vi "StopTrigger.vi"(8 "error in (no error)":errorcluster, 10 "trigger":string, 11 "PredictiveMaintenance in":refnum<class "PredictiveMaintenance.lvclass">) -> (0 "error out":errorcluster, 3 "PredictiveMaintenance out":refnum<class "PredictiveMaintenance.lvclass">)   [LabVIEW 2019, in "PredictiveMaintenance.lvlib" / "PredictiveMaintenance.lvclass"]
uses:
  PredictiveMaintenance.lvclass
  PredictiveMaintenance.lvclass/PredictiveMaintenance.ctl
  typedefs/Trigger_Data.ctl
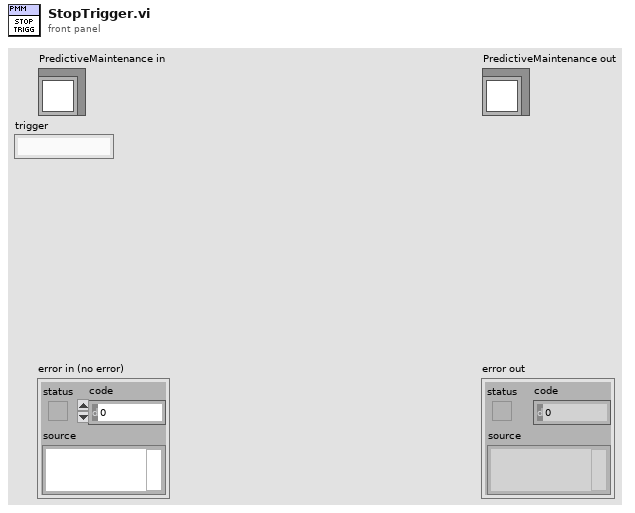
[diagram p1: front panel]
types:
  T1 = typedef "PredictiveMaintenance.lvlib/PredictiveMaintenance.lvclass/Trigger_Data.ctl" = cluster{"trigger":string, "curr_val (h)":dbl, "warn_limit (h)":dbl, "err_limit (h)":dbl, "running_timestamp":timestamp, "counter (h)":dbl}
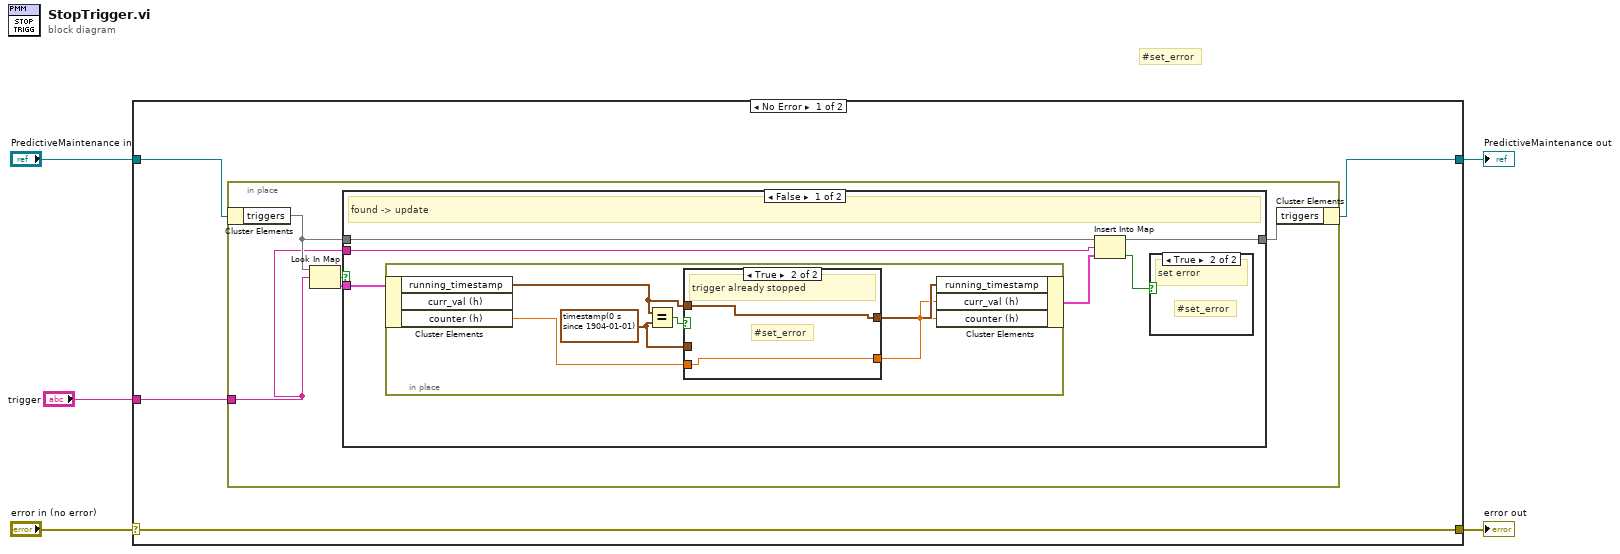
[diagram p0: block diagram]
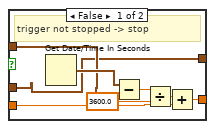
[diagram p3: hidden frame]
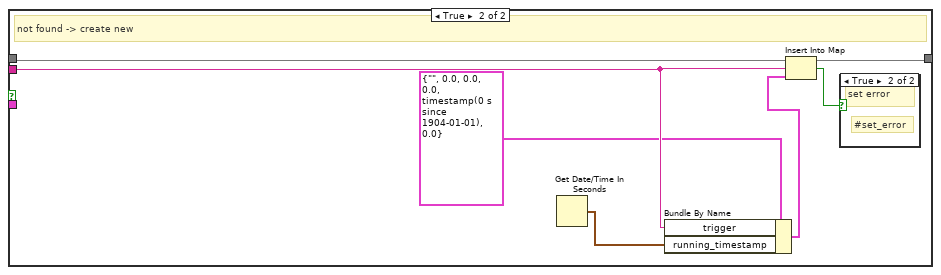
[diagram p4: hidden frame]
diagram:
  # "#set_error"
  n1 = case shown="No Error" "error in (no error)" {
    selector: "error in (no error)" -> [w9 w45]
    tunnel: [w9 w45] -> w4
    tunnel: [w7 w44] -> w2
    tunnel: "PredictiveMaintenance in" -> [w8 w44]
    tunnel: "trigger" -> [w6 _]
    frame No Error {
      n2 = in-place {
        in-place-border: w6 -> [w10]
        n3 = in-place-cluster #1(w8) -> ("triggers"=w13:map{string, T1})
        n4 = Look In Map(map=w13, key=w10) -> (key not found?=w14:bool, value=w12:T1)  [unwired: 1 in]
        n5 = case shown="False" w14 {
          tunnel: w13 -> [w20 w43]
          tunnel: w12 -> [w16 _]
          tunnel: [w19 w42] -> w11
          tunnel: w10 -> [w18 w41]
          frame False {
            # "found -> update"
            n6 = in-place {
              w23 = timestamp(0 s since 1904-01-01) ("current time")
              n7 = in-place-cluster #2(w16) -> ("running_timestamp"=w24:timestamp, "counter (h)"=w22:dbl)  [unwired: 1 out]
              n8 = Equal?(x=w24, y=w23) -> (x = y?=w26:bool)
              n9 = case shown="True" w26 {
                tunnel: [w27 w36] -> w25
                tunnel: w24 -> [w28 w36]
                tunnel: w23 -> [w27 _]
                tunnel: w22 -> [w31 w35]
                tunnel: [w29 w35] -> w21
                frame False {
                  # "trigger not stopped -> stop"
                  n10 = Get Date/Time In Seconds() -> (seconds since 1Jan1904=w34:timestamp)
                  n11 = Subtract(x=w34, y=w28) -> (x-y=w33:dbl)
                  n12 = Divide(x=w33, y=3600.0) -> (x/y=w32:dbl)
                  n13 = Add(x=w32, y=w31) -> (x+y=w29:dbl)
                }
                frame True {
                  # "#set_error"
                  # "trigger already stopped"
                }
              }
              n14 = in-place-cluster #2("running_timestamp"=w25, "curr_val (h)"=w21, "counter (h)"=w21) -> (w15:T1)
            }
            n15 = Insert Into Map(map in=w20, key=w18, value=w15) -> (map out=w19:map{string, T1}, value unchanged?=w17:bool)  [unwired: 1 out]
            n16 = case shown="True" w17 {
              frame False {
              }
              frame True {
                # "#set_error"
                # "set error"
              }
            }
          }
          frame True {
            # "not found -> create new"
            n17 = Get Date/Time In Seconds() -> (seconds since 1Jan1904=w38:timestamp)
            n18 = Bundle By Name(cluster=T1 {"trigger"="", "curr_val (h)"=0.0, "warn_limit (h)"=0.0, "err_limit (h)"=0.0, "running_timestamp"=timestamp(0 s since 1904-01-01), "counter (h)"=0.0} ("event_data"), "trigger"=w41, "running_timestamp"=w38) -> (w37:T1)
            n19 = Insert Into Map(map in=w43, key=w41, value=w37) -> (map out=w42:map{string, T1}, key already included?=w40:bool)  [unwired: 1 out]
            n20 = case shown="True" w40 {
              frame False {
              }
              frame True {
                # "#set_error"
                # "set error"
              }
            }
          }
        }
        n21 = in-place-cluster #1("triggers"=w11) -> (w7:refnum<class "PredictiveMaintenance.lvclass">)
      }
    }
    frame Error {
    }
  }
  "error out" <- w4
  "PredictiveMaintenance out" <- w2
